vi "Write FP Enable Items.vi"(10 "FP Enable Items":T1, 11 "FPEN":refnum<class "FPEN.lvclass">) -> (3 "FPEN Out":refnum<class "FPEN.lvclass">)   [LabVIEW 2025, in "FPEN.lvclass"]
uses:
  FPEN.lvclass
  TypeDefs_Utility/Cluster_FP_Show Hide Items.ctl
  TypeDefs_Utility/ENUM_FP_Show-Hide Select.ctl
  FPEN.lvclass/FPEN.ctl
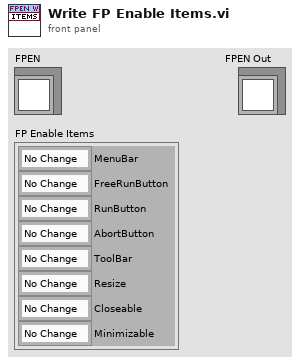
[diagram p1: front panel]
types:
  T1 = typedef "Cluster_FP_Show Hide Items.ctl" = cluster{"MenuBar":T2, "FreeRunButton":T2, "RunButton":T2, "AbortButton":T2, "ToolBar":T2, "Resize":T2, "Closeable":T2, "Minimizable":T2}
  T2 = typedef "ENUM_FP_Show-Hide Select.ctl" = enum16{"No Change", "Hide", "Show"}
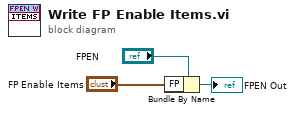
[diagram p0: block diagram]
diagram:
  n1 = Bundle By Name(cluster="FPEN", "FP"="FP Enable Items") -> (→"FPEN Out":refnum<class "FPEN.lvclass">)
